vi "Finish.vi"   [LabVIEW 2013]
doc: "This VI is called just before exiting. It is expected to close I/O refnum, save collected data, etc."
uses:
  <vilib>/Rock Robotics/WPI/Joystick/WPI_JoystickGetSetRefNum.vi
  <vilib>/Rock Robotics/WPI/RobotDrive/WPI_RobotDriveGetSetRefNum.vi
types:
  T1 = typedef "WPI_DigitalInputDevRef.ctl" = cluster{"DevStatus":errorcluster, "DIO Channel":T2, "Digital Module":T3}
  T2 = typedef "FPGA_DIOChannel.ctl" = enum8{"DIO 1", "DIO 2", "DIO 3", "DIO 4", "DIO 5", "DIO 6", "DIO 7", "DIO 8", "DIO 9", "DIO 10", "DIO 11", "DIO 12", "DIO 13", "DIO 14", "Invalid"}
  T3 = typedef "FPGA_TypedefDigitalModule.ctl" = enum16{"Digital Module 1", "Digital Module 2"}
  T4 = typedef "WPI_GyroDevRef.ctl" = cluster{"DevStatus":errorcluster, "Analog Module":T5, "Analog Channel":T6, "Offset":dbl, "Gain (VoltsPerDegree/Second)":dbl}
  T5 = typedef "FPGA_TypedefAnalogModule.ctl" = enum16{"Analog Module 1", "Analog Module 2"}
  T6 = typedef "FPGA_AIChannel.ctl" = enum8{"AI 1", "AI 2", "AI 3", "AI 4", "AI 5", "AI 6", "AI 7", "AI 8", "Invalid"}
  T7 = typedef "WPI_AnalogChannelDevRef.ctl" = cluster{"DevStatus":errorcluster, "Analog Module":T5, "Analog Channel":T6}
  T8 = typedef "WPI_EncoderDevRef.ctl" = cluster{"DevStatus":errorcluster, "EncoderIndex":T9, "CounterIndex":T10, "DistancePerCount":dbl, "Decoding Type":T11}
  T9 = typedef "FPGA_EncoderIdx.ctl" = enum8{"Enc 0", "Enc 1", "Enc 2", "Enc 3", "Invalid"}
  T10 = typedef "FPGA_CounterCtrSystemIndex.ctl" = enum8{"Ctr 0", "Ctr 1", "Ctr 2", "Ctr 3", "Ctr 4", "Ctr 5", "Ctr 6", "Ctr 7", "Invalid"}
  T11 = typedef "WPI_EncoderType.ctl" = enum16{"1x", "2x", "4x"}
  T12 = typedef "WPI_CounterDevRef.ctl" = cluster{"DevStatus":errorcluster, "CntIndex":T10}
  T13 = typedef "WPI_SolenoidDevRef.ctl" = cluster{"DevStatus":errorcluster, "Solenoid Module":T14, "Forward Solenoid Channel":T15, "Reverse Solenoid Channel":T15}
  T14 = typedef "FPGA_TypedefSolenoidModule.ctl" = enum16{"Solenoid Module 1", "Solenoid Module 2"}
  T15 = typedef "WPI_SolenoidChannel.ctl" = enum8{"Solenoid 1", "Solenoid 2", "Solenoid 3", "Solenoid 4", "Solenoid 5", "Solenoid 6", "Solenoid 7", "Solenoid 8", "Invalid"}
  T16 = typedef "WPI_CameraDevRef.ctl" = cluster{"Camera Address":string, "CameraStatus":errorcluster, "Acquire Image Notifier":refnum<notifier>}
  T17 = typedef "WPI_JoystickDevRef.ctl" = cluster{"Device":T18}
  T18 = typedef "WPI_JoystickDeviceEnum.ctl" = enum16{"USB 1", "USB 2", "USB 3", "USB 4", "Kinect 1", "Kinect 2"}
  T19 = typedef "WPI_MotorControlDeviceRef.ctl" = cluster{"DeviceStatus":errorcluster, "Type":enum16{"PWM", "CAN"}, "PWM":cluster{"Digital Module":T3, "PWM Channel":T20, "DeadBand":T21}, "CAN":cluster{"Device Number":u8, "Control Mode":T22, "Semaphore":T23, "Max Vout":dbl}, "Invert":bool, "TransformRef":T24, "InvTransformRef":T24}
  T20 = typedef "FPGA_DIOPWMChannel.ctl" = enum8{"PWM 1", "PWM 2", "PWM 3", "PWM 4", "PWM 5", "PWM 6", "PWM 7", "PWM 8", "PWM 9", "PWM 10", "Invalid"}
  T21 = typedef "WPI_PWMDeadband.ctl" = cluster{"Name":string, "maxPositivePwm":i32, "minPositivePwm":i32, "centerPwm":i32, "maxNegativePwm":i32, "minNegativePwm":i32, "angularRange":u16}
  T22 = typedef "WPI_CANJaguar_ControlMode.ctl" = enum8{"Percent VBus", "Current", "Speed", "Position", "Voltage"}
  T23 = typedef "Semaphore RefNum" = refnum<k1>
  T24 = typedef "WPI_PWMTransform_ConPane.ctl" = refnum<vi>
  T25 = typedef "WPI_RobotDriveDevRef.ctl" = cluster{"DevStatus":errorcluster, "Motors[]":T19[], "Square Inputs":bool, "Max Output":dbl, "Isochronous":bool}
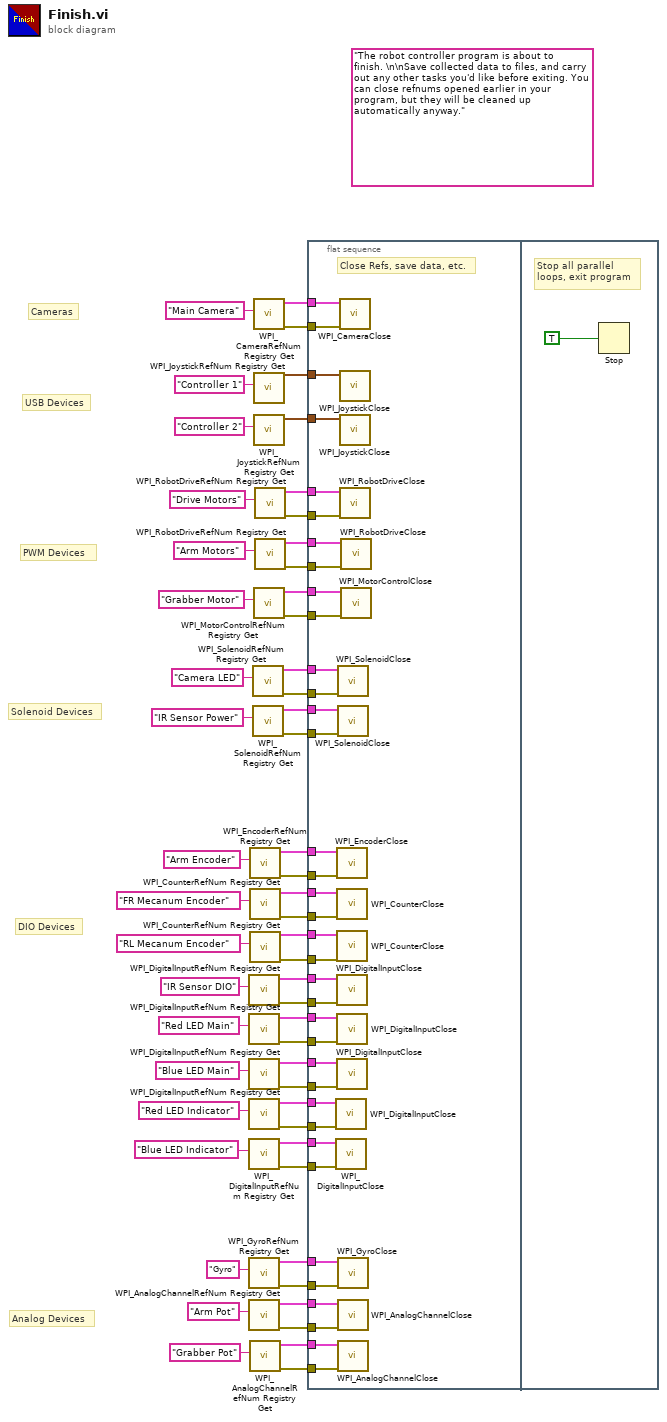
[diagram p0: block diagram]
diagram:
  (unwired) "The robot controller program is about to finish. \n\nSave collected data to files, and carry out any other tasks you'd like before exiting. You can close refnums opened earlier in your program, but they will be cleaned up automatically anyway."
  # "Analog Devices"
  # "DIO Devices"
  # "Cameras"
  # "Solenoid Devices"
  # "PWM Devices"
  # "USB Devices"
  n1 = call <vilib>:"WPI_DigitalInputRefNum Registry Get.vi"("refnum name"="IR Sensor DIO") -> ("error out"=w18:errorcluster, "DigitalInputDevRef"=w19:T1)  [unwired: 9 in]
  n2 = call <vilib>:"WPI_DigitalInputRefNum Registry Get.vi"("refnum name"="Red LED Main") -> ("error out"=w13:errorcluster, "DigitalInputDevRef"=w14:T1)  [unwired: 9 in]
  n3 = call <vilib>:"WPI_DigitalInputRefNum Registry Get.vi"("refnum name"="Blue LED Main") -> ("error out"=w8:errorcluster, "DigitalInputDevRef"=w9:T1)  [unwired: 9 in]
  n4 = call <vilib>:"WPI_DigitalInputRefNum Registry Get.vi"("refnum name"="Red LED Indicator") -> ("error out"=w6:errorcluster, "DigitalInputDevRef"=w5:T1)  [unwired: 9 in]
  n5 = call <vilib>:"WPI_DigitalInputRefNum Registry Get.vi"("refnum name"="Blue LED Indicator") -> ("error out"=w4:errorcluster, "DigitalInputDevRef"=w7:T1)  [unwired: 9 in]
  n6 = call <vilib>:"WPI_GyroRefNum Registry Get.vi"("refnum name"="Gyro") -> ("error out"=w29:errorcluster, "GyroDevRef"=w30:T4)  [unwired: 9 in]
  n7 = call <vilib>:"WPI_AnalogChannelRefNum Registry Get.vi"("refnum name"="Arm Pot") -> ("error out"=w21:errorcluster, "AIDeviceRef"=w28:T7)  [unwired: 9 in]
  n8 = call <vilib>:"WPI_EncoderRefNum Registry Get.vi"("refnum name"="Arm Encoder") -> ("error out"=w1:errorcluster, "EncoderDevRef"=w2:T8)  [unwired: 9 in]
  n9 = call <vilib>:"WPI_CounterRefNum Registry Get.vi"("refnum name"="FR Mecanum Encoder") -> ("error out"=w22:errorcluster, "CounterDevRef"=w35:T12)  [unwired: 9 in]
  n10 = call <vilib>:"WPI_CounterRefNum Registry Get.vi"("refnum name"="RL Mecanum Encoder") -> ("error out"=w23:errorcluster, "CounterDevRef"=w34:T12)  [unwired: 9 in]
  n11 = call <vilib>:"WPI_AnalogChannelRefNum Registry Get.vi"("refnum name"="Grabber Pot") -> ("error out"=w20:errorcluster, "AIDeviceRef"=w27:T7)  [unwired: 9 in]
  n12 = call <vilib>:"WPI_SolenoidRefNum Registry Get.vi"("refnum name"="Camera LED") -> ("error out"=w16:errorcluster, "SolenoidDevRef"=w42:T13)  [unwired: 9 in]
  n13 = call <vilib>:"WPI_SolenoidRefNum Registry Get.vi"("refnum name"="IR Sensor Power") -> ("error out"=w24:errorcluster, "SolenoidDevRef"=w40:T13)  [unwired: 9 in]
  n14 = call <vilib>:"WPI_CameraRefNum Registry Get.vi"("refnum name"="Main Camera") -> ("error out"=w37:errorcluster, "CameraDevRef"=w38:T16)  [unwired: 9 in]
  n15 = call <vilib>:"WPI_JoystickRefNum Registry Get.vi"("refnum name"="Controller 1") -> ("JoystickDevRef"=w46:T17)  [unwired: 9 in, 1 out]
  n16 = call <vilib>:"WPI_JoystickRefNum Registry Get.vi"("refnum name"="Controller 2") -> ("JoystickDevRef"=w43:T17)  [unwired: 9 in, 1 out]
  n17 = call <vilib>:"WPI_MotorControlRefNum Registry Get.vi"("refnum name"="Grabber Motor") -> ("error out"=w48:errorcluster, "MotorControlDevRef"=w49:T19)  [unwired: 9 in]
  n18 = call <vilib>:"WPI_RobotDriveRefNum Registry Get.vi"("refnum name"="Drive Motors") -> ("error out"=w53:errorcluster, "RobotDriveDevRef"=w54:T25)  [unwired: 9 in]
  n19 = call <vilib>:"WPI_RobotDriveRefNum Registry Get.vi"("refnum name"="Arm Motors") -> ("error out"=w51:errorcluster, "RobotDriveDevRef"=w52:T25)  [unwired: 9 in]
  n20 = flat-sequence {
    tunnel: w54 -> [w91]
    tunnel: w53 -> [w90]
    tunnel: w52 -> [w89]
    tunnel: w51 -> [w88]
    tunnel: w49 -> [w87]
    tunnel: w48 -> [w86]
    tunnel: w46 -> [w85]
    tunnel: w43 -> [w84]
    tunnel: w42 -> [w83]
    tunnel: w40 -> [w82]
    tunnel: w38 -> [w81]
    tunnel: w37 -> [w80]
    tunnel: w35 -> [w79]
    tunnel: w34 -> [w78]
    tunnel: w30 -> [w77]
    tunnel: w29 -> [w76]
    tunnel: w28 -> [w75]
    tunnel: w27 -> [w74]
    tunnel: w24 -> [w73]
    tunnel: w23 -> [w72]
    tunnel: w22 -> [w71]
    tunnel: w21 -> [w70]
    tunnel: w20 -> [w69]
    tunnel: w19 -> [w68]
    tunnel: w18 -> [w67]
    tunnel: w16 -> [w66]
    tunnel: w14 -> [w65]
    tunnel: w13 -> [w64]
    tunnel: w9 -> [w63]
    tunnel: w8 -> [w62]
    tunnel: w7 -> [w61]
    tunnel: w6 -> [w60]
    tunnel: w5 -> [w59]
    tunnel: w4 -> [w58]
    tunnel: w2 -> [w57]
    tunnel: w1 -> [w56]
    frame #0 {
      # "Close Refs, save data, etc."
      n21 = call <vilib>:"WPI_DigitalInputClose.vi"("error in (no error)"=w60, "DigitalInputDevRef"=w59) -> ()  [unwired: 9 in, 1 out]
      n22 = call <vilib>:"WPI_DigitalInputClose.vi"("error in (no error)"=w58, "DigitalInputDevRef"=w61) -> ()  [unwired: 9 in, 1 out]
      n23 = call <vilib>:"WPI_EncoderClose.vi"("error in (no error)"=w56, "EncoderDevRef"=w57) -> ()  [unwired: 9 in, 1 out]
      n24 = call <vilib>:"WPI_CounterClose.vi"("error in (no error)"=w71, "CounterDevRef"=w79) -> ()  [unwired: 9 in, 1 out]
      n25 = call <vilib>:"WPI_CounterClose.vi"("error in (no error)"=w72, "CounterDevRef"=w78) -> ()  [unwired: 9 in, 1 out]
      n26 = call <vilib>:"WPI_DigitalInputClose.vi"("error in (no error)"=w67, "DigitalInputDevRef"=w68) -> ()  [unwired: 9 in, 1 out]
      n27 = call <vilib>:"WPI_DigitalInputClose.vi"("error in (no error)"=w64, "DigitalInputDevRef"=w65) -> ()  [unwired: 9 in, 1 out]
      n28 = call <vilib>:"WPI_DigitalInputClose.vi"("error in (no error)"=w62, "DigitalInputDevRef"=w63) -> ()  [unwired: 9 in, 1 out]
      n29 = call <vilib>:"WPI_SolenoidClose.vi"("error in (no error)"=w66, "SolenoidDevRef"=w83) -> ()  [unwired: 9 in, 1 out]
      n30 = call <vilib>:"WPI_SolenoidClose.vi"("error in (no error)"=w73, "SolenoidDevRef"=w82) -> ()  [unwired: 9 in, 1 out]
      n31 = call <vilib>:"WPI_GyroClose.vi"("error in (no error)"=w76, "GyroDevRef"=w77) -> ()  [unwired: 9 in, 1 out]
      n32 = call <vilib>:"WPI_AnalogChannelClose.vi"("error in (no error)"=w70, "AIDeviceRef"=w75) -> ()  [unwired: 9 in, 1 out]
      n33 = call <vilib>:"WPI_AnalogChannelClose.vi"("error in (no error)"=w69, "AIDeviceRef"=w74) -> ()  [unwired: 9 in, 1 out]
      n34 = call <vilib>:"WPI_CameraClose.vi"("error in (no error)"=w80, "CameraDevRef"=w81) -> ()  [unwired: 9 in, 1 out]
      n35 = call <vilib>:"WPI_JoystickClose.vi"("JoystickDevRef"=w85) -> ()  [unwired: 11 in]
      n36 = call <vilib>:"WPI_JoystickClose.vi"("JoystickDevRef"=w84) -> ()  [unwired: 11 in]
      n37 = call <vilib>:"WPI_RobotDriveClose.vi"("error in (no error)"=w90, "RobotDriveDevRef"=w91) -> ()  [unwired: 9 in, 1 out]
      n38 = call <vilib>:"WPI_RobotDriveClose.vi"("error in (no error)"=w88, "RobotDriveDevRef"=w89) -> ()  [unwired: 9 in, 1 out]
      n39 = call <vilib>:"WPI_MotorControlClose.vi"("error in (no error)"=w86, "MotorControlDevRef"=w87) -> ()  [unwired: 9 in, 1 out]
    }
    frame #1 {
      # "Stop all parallel\nloops, exit program"
      n40 = Stop(stop? (T)=TRUE ("Quit")) -> ()
    }
  }
